vi "Dynamic Results Status Update Process.vi"(8 "error in (no error)":errorcluster, 10 "TestStatusEvents":T1, 11 "TestRunner_UI_Refs":T2) -> (0 "error out":errorcluster)   [LabVIEW 2011, in "GraphicalTestRunner.lvlib"]
uses:
  GraphicalTestRunner.lvlib
  Classes/TestResult/resultStatus--enum.ctl
  Classes/TestResult/TestResult.lvclass
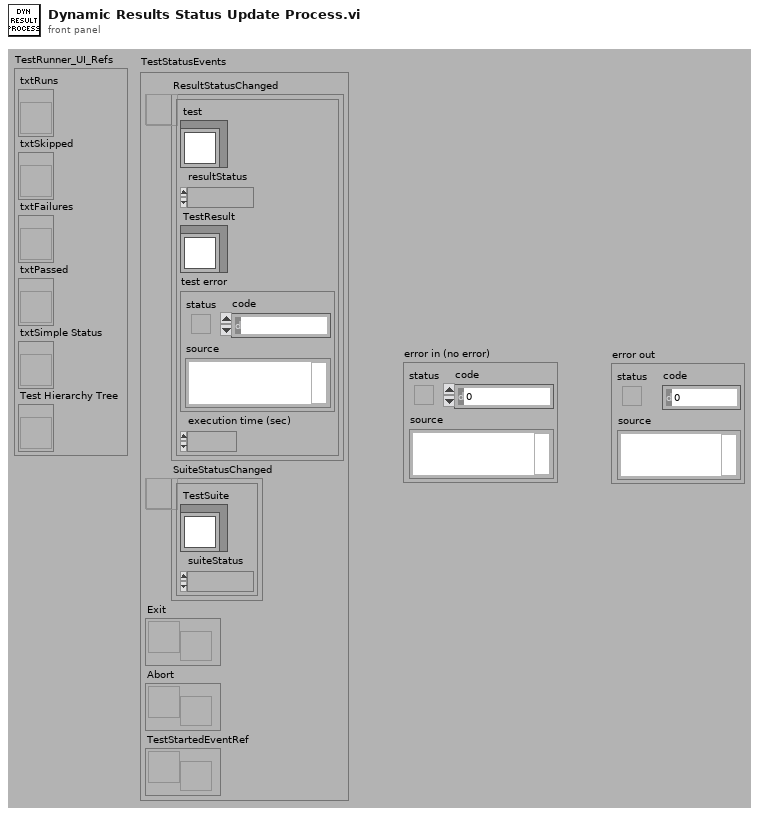
[diagram p1: front panel]
types:
  T1 = cluster{"ResultStatusChanged":refnum<user-event>, "SuiteStatusChanged":refnum<user-event>, "Exit":refnum<user-event>, "Abort":refnum<user-event>, "TestStartedEventRef":refnum<user-event>}
  T2 = cluster{"txtRuns":refnum<vi>, "txtSkipped":refnum<vi>, "txtFailures":refnum<vi>, "txtPassed":refnum<vi>, "txtSimple Status":refnum<vi>, "Test Hierarchy Tree":refnum<vi>}
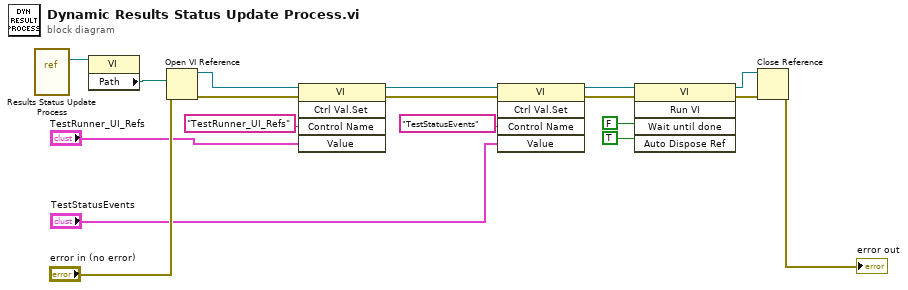
[diagram p0: block diagram]
diagram:
  n1 = vi-ref "Results Status Update Process.vi"() -> (w16:refnum<vi>)
  n2 = property class="VI"(reference=w16) -> ("Path"=w18:path)  [unwired: 1 in, 2 out]
  n3 = Open VI Reference(vi path=w18, error in (no error)="error in (no error)") -> (vi reference=w13:refnum<vi>, error out=w12:errorcluster)  [unwired: 4 in]
  n4 = invoke class="VI" method="Ctrl Val.Set"(reference=w13, error in=w12, "Control Name"="TestRunner_UI_Refs", "Value"="TestRunner_UI_Refs") -> (reference out=w7:refnum<vi>, error out=w11:errorcluster)  [unwired: 1 in, 3 out]
  n5 = invoke class="VI" method="Ctrl Val.Set"(reference=w7, error in=w11, "Control Name"="TestStatusEvents", "Value"="TestStatusEvents") -> (reference out=w6:refnum<vi>, error out=w10:errorcluster)  [unwired: 1 in, 3 out]
  n6 = invoke class="VI" method="Run VI"(reference=w6, error in=w10, "Wait until done"=FALSE, "Auto Dispose Ref"=TRUE) -> (reference out=w5:refnum<vi>, error out=w9:errorcluster)  [unwired: 1 in, 3 out]
  n7 = Close Reference(reference=w5, error in (no error)=w9) -> (error out=→"error out":errorcluster)
